vi "Thermistor-ConversionV2.vi"(0 "Resistor":dbl, 1 "A":dbl, 2 "B":dbl, 3 "Input voltage":dbl=5.04 format="%#_13g", 4 "Sensor Voltage":dbl, 5 "C":dbl) -> (6 "Temp":dbl)   [LabVIEW 2020]
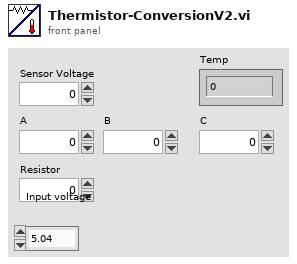
[diagram p1: front panel]
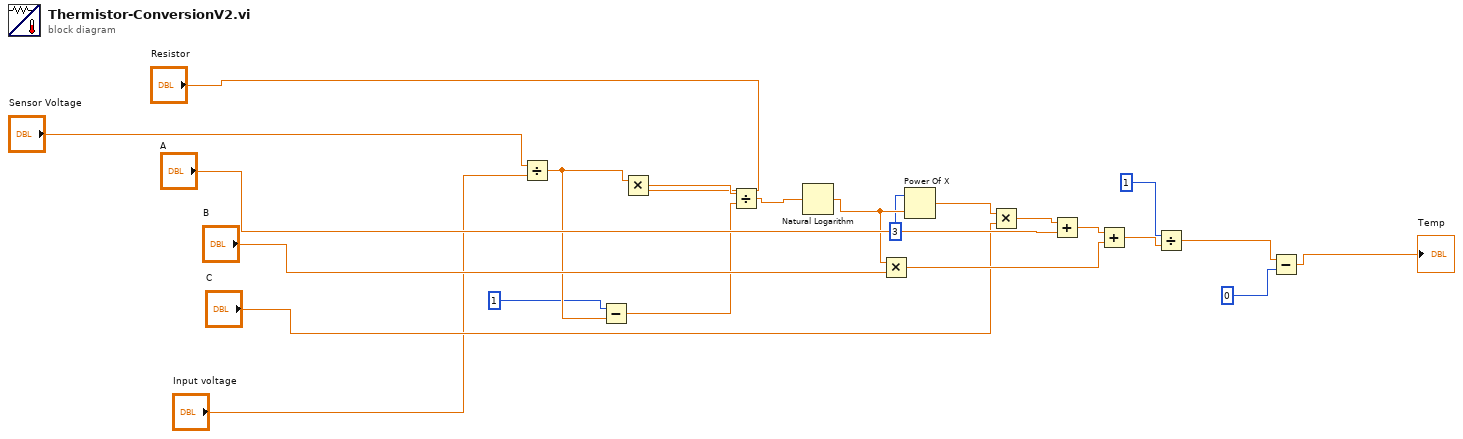
[diagram p0: block diagram]
diagram:
  n1 = Divide(x="Sensor Voltage", y="Input voltage") -> (x/y=w6:dbl)
  n2 = Subtract(x=1, y=w6) -> (x-y=w7:dbl)
  n3 = Multiply(x=w6, y="Resistor") -> (x*y=w4:dbl)
  n4 = Divide(x=w4, y=w7) -> (x/y=w22:dbl)
  n5 = Natural Logarithm(1:w22) -> (0:w11:dbl)
  n6 = Multiply(x=w11, y="B") -> (x*y=w16:dbl)
  n7 = Power Of X(1:w11, 2:3) -> (0:w9:dbl)
  n8 = Multiply(x=w9, y="C") -> (x*y=w13:dbl)
  n9 = Add(x=w13, y="A") -> (x+y=w15:dbl)
  n10 = Add(x=w15, y=w16) -> (x+y=w17:dbl)
  n11 = Divide(x=1, y=w17) -> (x/y=w19:dbl)
  n12 = Subtract(x=w19, y=0) -> (x-y=→"Temp":dbl)
